vi "Calculate Wavelength v0.3.vi"(3 "pixel index":dbl=512.0 min=0.0 max=1024.0 format="%.2f", 4 "Current Grating Density":enum16{"150", "300", "600", "1200", "1800"}(ring)=enum."600" caption="Grating Density", 5 "Central Wavelength":dbl=600.0 format="%.2f") -> (1 "nm (out)":dbl=571.2504622529284 format="%.4f")   [LabVIEW 2020]
panel:
  out "Detector Pixel Distance":dbl=27.0 format="%.2f"
  out "beta":dbl=0.03851514953863218 format="%.2f"
  out "alpha":dbl=21.141484850461367 format="%.2f"
  out "Spectrometer Mirror angle":dbl=21.18 format="%.2f"
  out "Spectrometer Focal length":dbl=750.0 format="%.1f"
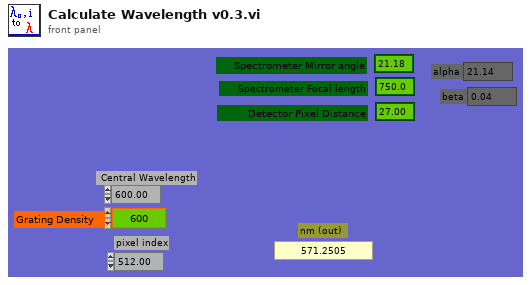
[diagram p1: front panel]
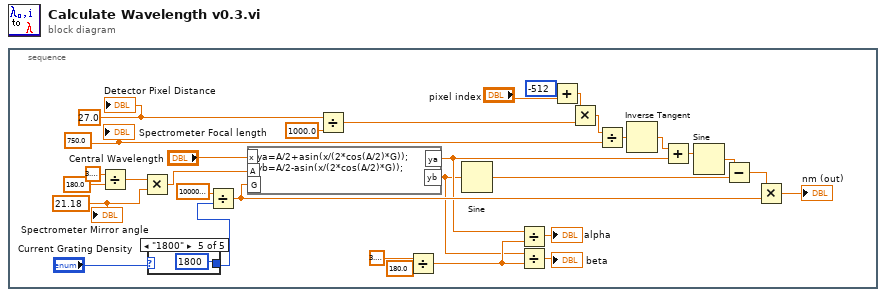
[diagram p0: block diagram]
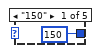
[diagram p2: hidden frame]
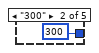
[diagram p3: hidden frame]
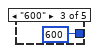
[diagram p4: hidden frame]
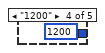
[diagram p5: hidden frame]
diagram:
  n1 = stacked-sequence {
    frame #0 {
      w25 = 21.18 ("Detector Pixel Distance")
      w24 = 750.0 ("Detector Pixel Distance")
      w26 = 27.0 ("x")
      n2 = Divide(x=3.141592653589793, y=180.0) -> (x/y=w18:dbl)
      n3 = Multiply(x=w18, y=w25) -> (x*y=w23:dbl)
      n4 = case shown="\"1800\"" "Current Grating Density" {
        tunnel: [150 300 600 1200 1800] -> w12
        frame "150" {
        }
        frame "300" {
        }
        frame "600" {
        }
        frame "1200" {
        }
        frame "1800" {
        }
      }
      n5 = Divide(x=1000000.0, y=w12) -> (x/y=w22:dbl)
      n6 = formula code="ya=A/2+asin(x/(2*cos(A/2)*G));\nyb=A/2-asin(x/(2*cos(A/2)*G));"("x"="Central Wavelength", "A"=w23, "G"=w22) -> ("ya"=w16:dbl, "yb"=w15:dbl)
      n7 = Divide(x=w26, y=1000.0) -> (x/y=w28:dbl)
      n8 = Divide(x=3.141592653589793, y=180.0) -> (x/y=w21:dbl)
      n9 = Sine(x=w15) -> (sin(x)=w27:dbl)
      n10 = Divide(x=w16, y=w21) -> (x/y=→"alpha":dbl)
      n11 = Divide(x=w15, y=w21) -> (x/y=→"beta":dbl)
      n12 = Add(x=-512, y="pixel index") -> (x+y=w3:dbl)
      n13 = Multiply(x=w3, y=w28) -> (x*y=w5:dbl)
      n14 = Divide(x=w5, y=w24) -> (x/y=w8:dbl)
      n15 = Inverse Tangent(1:w8) -> (0:w7:dbl)
      n16 = Add(x=w7, y=w16) -> (x+y=w6:dbl)
      n17 = Sine(x=w6) -> (sin(x)=w10:dbl)
      n18 = Subtract(x=w10, y=w27) -> (x-y=w9:dbl)
      n19 = Multiply(x=w9, y=w22) -> (x*y=→"nm (out)":dbl)
      "Spectrometer Focal length" <- w24
      "Spectrometer Mirror angle" <- w25
      "Detector Pixel Distance" <- w26
    }
  }
